vi "Run.vi"(8 "error in (no error)":errorcluster caption="entrée d'erreur (pas d'erreur)", 10 "X":string[][](array[string]), 11 "robust_scale.lvclass":refnum<class "robust_scale.lvclass">) -> (0 "error out":errorcluster caption="sortie d'erreur", 2 "Data":T1, 3 "robust_scale.lvclass":refnum<class "robust_scale.lvclass">)   [LabVIEW 2020, in "robust_scale.lvclass"]
uses:
  robust_scale.lvclass
  robust_scale.lvclass/robust_scale.ctl
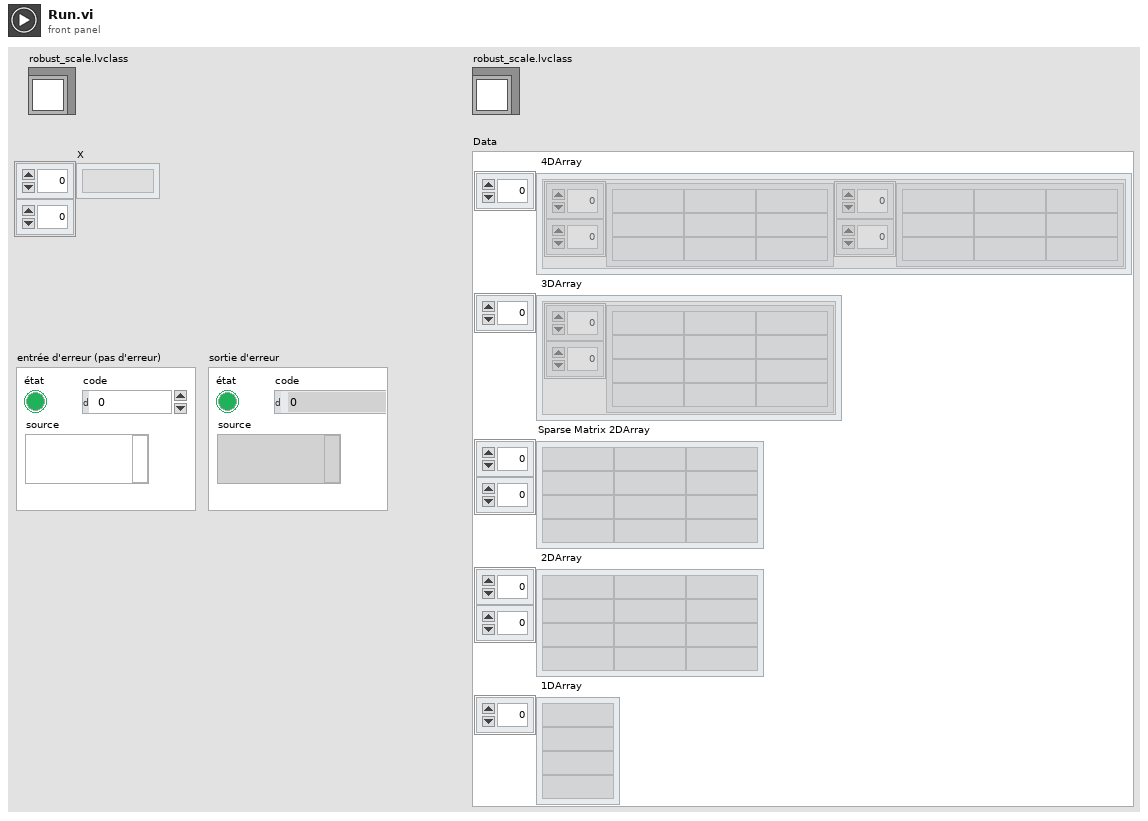
[diagram p1: front panel]
types:
  T1 = cluster{" 4DArray":cluster{"1":string[][], "2":string[][]}[], " 3DArray":cluster{"Tableau":string[][]}[], "Sparse Matrix 2DArray":string[][], " 2DArray":string[][], " 1DArray":string[]}
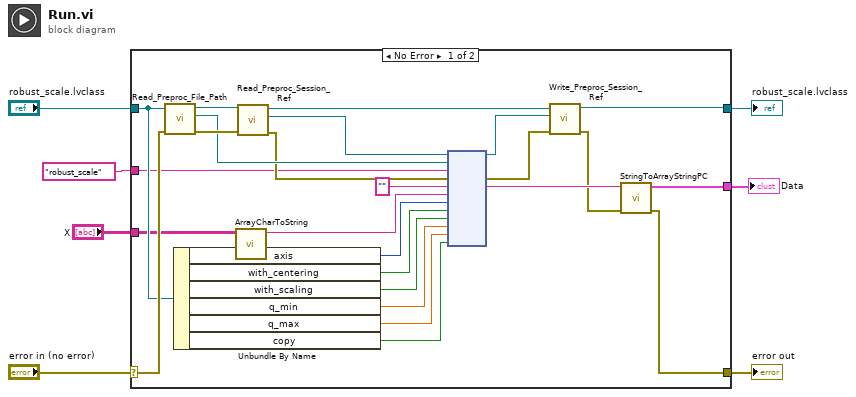
[diagram p0: block diagram]
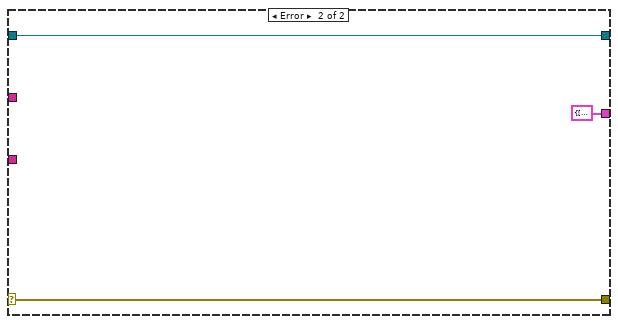
[diagram p2: hidden frame]
diagram:
  n1 = case shown="No Error" "error in (no error)" {
    selector: "error in (no error)" -> [w21 w35]
    tunnel: [w9 w35] -> w6
    tunnel: [w11 w34] -> w4
    tunnel: "robust_scale.lvclass" -> [w20 w34]
    tunnel: "robust_scale" ("Fonction") -> [w19 _]
    tunnel: [w8 T1 {" 4DArray"=[], " 3DArray"=[], "Sparse Matrix 2DArray"=[], " 2DArray"=[], " 1DArray"=[]} ("Data")] -> w1
    tunnel: "X" -> [w14 _]
    frame No Error {
      n2 = call-dynamic "Read_Preproc_File_Path.vi"("error in (no error)"=w21, "Python in"=w20) -> ("error out"=w31:errorcluster, "File_Path"=w28:path, "Python out"=w32:refnum<class "robust_scale.lvclass">)  [unwired: 7 in]
      n3 = Unbundle By Name(w20) -> ("axis"=w23:i32, "with_centering"=w22:bool, "with_scaling"=w18:bool, "q_min"=w17:dbl, "q_max"=w16:dbl, "copy"=w15:bool)
      n4 = call "ArrayCharToString.vi"("TAB"=w14) -> ("Instruction"=w13:string)  [unwired: 10 in]
      n5 = call-dynamic "Read_Preproc_Session_Ref.vi"("error in (no error)"=w31, "Python in"=w32) -> ("error out"=w27:errorcluster, "Session_ref"=w29:refnum<k35>, "Python out"=w30:refnum<class "robust_scale.lvclass">)  [unwired: 7 in]
      n6 = node(w29, w28, w19, w27, "", w13, w23, w22, w18, w17, w16, w15) -> (w25:refnum<k35>, w26:errorcluster, w12:string)  [unwired: 7 in, 2 out]
      n7 = call-dynamic "Write_Preproc_Session_Ref.vi"("error in (no error)"=w26, "Session_ref"=w25, "Python in"=w30) -> ("error out"=w10:errorcluster, "Python out"=w11:refnum<class "robust_scale.lvclass">)  [unwired: 7 in]
      n8 = call "StringToArrayStringPC.vi"("sortie d'erreur"=w10, "Return value"=w12) -> ("sortie d'erreur"=w9:errorcluster, "Data"=w8:T1)  [unwired: 8 in]
    }
    frame Error {
    }
  }
  "error out" <- w6
  "robust_scale.lvclass" <- w4
  "Data" <- w1
